vi "Set Ctl Value.vi"(8 "error in (no error)":errorcluster, 9 "Signaling?":bool, 10 "String":string, 11 "Numeric Field in":refnum<class "Numeric Field.lvclass">) -> (0 "error out":errorcluster, 3 "Numeric Field out":refnum<class "Numeric Field.lvclass">)   [LabVIEW 2020, in "Old Basic Fields.lvlib" / "Numeric Field.lvclass"]
uses:
  Numeric Field.lvclass
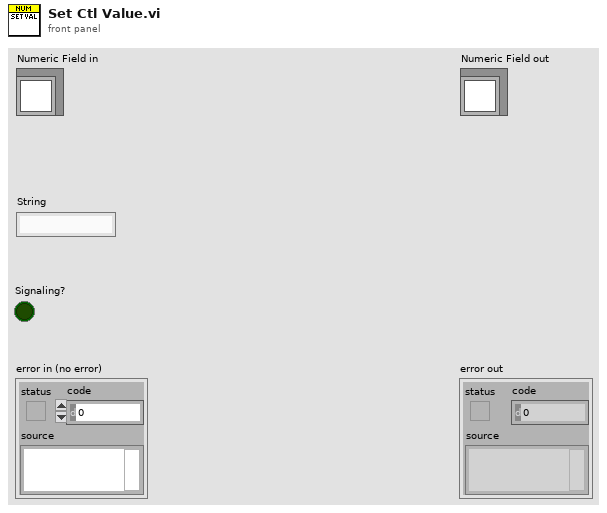
[diagram p1: front panel]
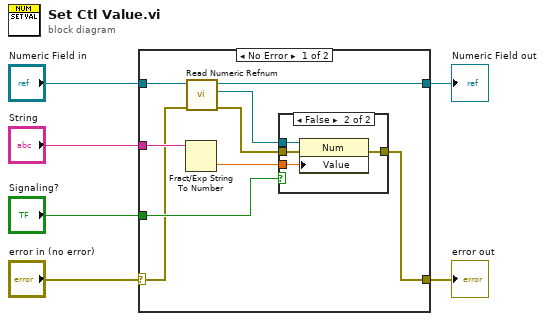
[diagram p0: block diagram]
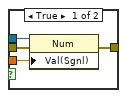
[diagram p2: hidden frame]
diagram:
  n1 = case shown="No Error" "error in (no error)" {
    selector: "error in (no error)" -> [w7 w25]
    tunnel: [w9 w25] -> w5
    tunnel: "Numeric Field in" -> [w15 w24]
    tunnel: [w14 w24] -> w3
    tunnel: "String" -> [w13 _]
    tunnel: "Signaling?" -> [w10 _]
    frame No Error {
      n2 = Fract/Exp String To Number(string=w13) -> (number=w11:dbl)  [unwired: 3 in, 1 out]
      n3 = call "Read Numeric Refnum.vi"("error in (no error)"=w7, "Numeric Field in"=w15) -> ("error out"=w8:errorcluster, "Num Refnum"=w12:refnum<vi>, "Numeric Field out"=w14:refnum<class "Numeric Field.lvclass">)  [unwired: 7 in]
      n4 = case shown="False" w10 {
        tunnel: w12 -> [w19 w23]
        tunnel: w11 -> [w18 w22]
        tunnel: [w17 w21] -> w9
        tunnel: w8 -> [w16 w20]
        frame True {
          n5 = property class="Num"(reference=w19, error in=w16, "Val(Sgnl)"=w18) -> (error out=w17:errorcluster)  [unwired: 1 out]
        }
        frame False {
          n6 = property class="Num"(reference=w23, error in=w20, "Value"=w22) -> (error out=w21:errorcluster)  [unwired: 1 out]
        }
      }
    }
    frame Error {
    }
  }
  "error out" <- w5
  "Numeric Field out" <- w3
